vi "Write Parent State.vi"(8 "error in (no error)":errorcluster, 10 "Parent State":refnum<class "_State Machine Actor.lvclass">, 11 "State Machine Actor in":refnum<class "State Machine Actor.lvclass">) -> (0 "error out":errorcluster, 3 "State Machine Actor out":refnum<class "State Machine Actor.lvclass">)   [LabVIEW 2024, in "State Machine Actor.lvlib" / "State Machine Actor.lvclass"]
uses:
  State Machine Actor.lvclass
  State Machine Actor.lvclass/State Machine Actor.ctl
  _State Machine Actor/_State Machine Actor/_State Machine Actor.lvclass
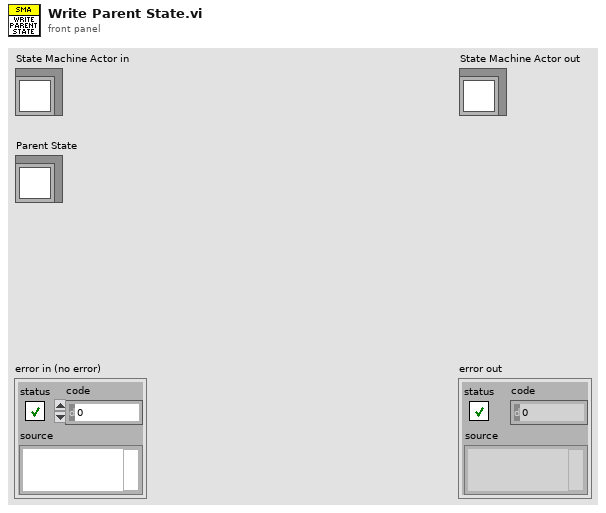
[diagram p1: front panel]
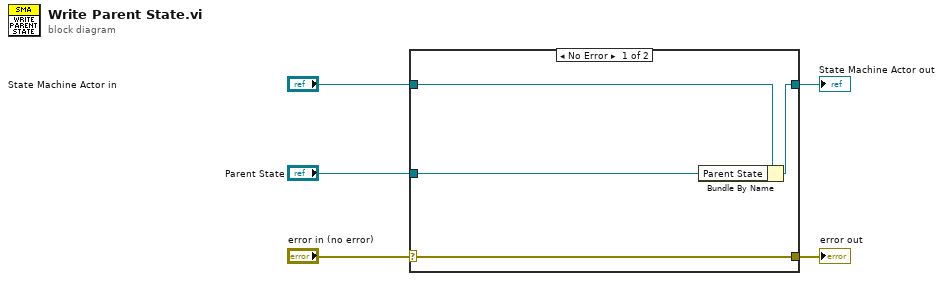
[diagram p0: block diagram]
diagram:
  n1 = case shown="No Error" "error in (no error)" {
    selector: "error in (no error)" -> [w9 w10]
    tunnel: [w9 w10] -> w4
    tunnel: [w7 w11] -> w2
    tunnel: "State Machine Actor in" -> [w8 w11]
    tunnel: "Parent State" -> [w6 _]
    frame No Error {
      n2 = Bundle By Name(cluster=w8, "Parent State"=w6) -> (w7:refnum<class "State Machine Actor.lvclass">)
    }
    frame Error {
    }
  }
  "error out" <- w4
  "State Machine Actor out" <- w2
